vi "Title-Get.vi"(8 "error in (no error)":errorcluster, 11 "WindowBuilder in":refnum<class "WindowBuilder.lvclass">) -> (0 "error out":errorcluster, 2 "Title":string, 3 "WindowBuilder out":refnum<class "WindowBuilder.lvclass">)   [LabVIEW 2024, in "GLF.lvlib" / "WindowBuilder.lvclass"]
uses:
  WindowBuilder.lvclass
  WindowBuilder.lvclass/WindowBuilder.ctl
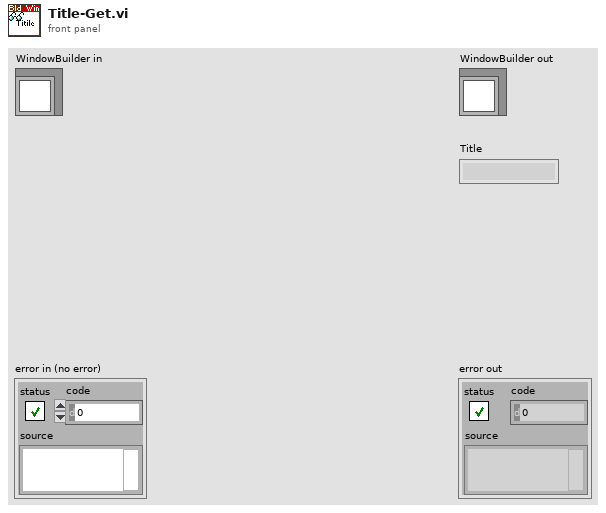
[diagram p1: front panel]
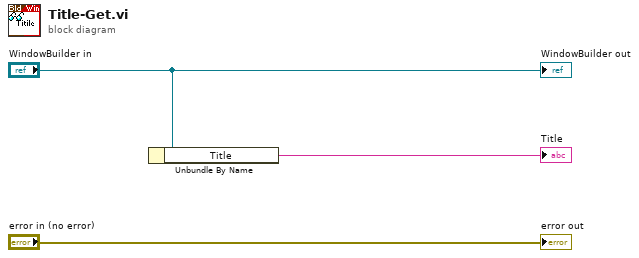
[diagram p0: block diagram]
diagram:
  n1 = Unbundle By Name("WindowBuilder in") -> ("Title"=→"Title":string)
  "error out" <- "error in (no error)"
  "WindowBuilder out" <- "WindowBuilder in"
